vi "Vision Tracking.vi"(0 "Color Image In":T4, 1 "Score Limits":T7={"Rect Coverage"=76.0, "Aspect Ratio"=70.0, "X Edge Strength"=40.0, "Y Edge Strength"=60.0}, 3 "Decimate by":cluster{"H":i32, "V":i32}={"H"=3, "V"=5}, 4 "Color Range":T8={"Hue"={"Lower"=55, "Upper"=93}, "Sat"={"Lower"=41, "Upper"=255}, " Luma"={"Lower"=99, "Upper"=255}}, 5 "Left Offset Percentage":dbl=3.0, 6 "Camera Type":enum16{"206", "1011"}(ring), 9 "Particle Count Limit":i32=10, 11 "Display Mask":bool, 12 "Image Size":T6=enum."320x240", 13 "Area Size Limit":i32=444) -> (14 "Processed Image":T4, 15 "Distance (ft)":dbl, 17 "Target Info":T5(array[cluster]), 18 "Position.X":dbl, 19 "Center Line X":dbl)   [LabVIEW 2011]
uses:
  <vilib>/vision/Image Controls.llb/IMAQ Image.ctl
  <vilib>/Rock Robotics/WPI/Camera/WPI_CameraImageSize.ctl
  <vilib>/addons/control/pid/NI_PID_pid.lvlib
panel:
  out "Top Goal Left and Right":cluster{"Left":dbl, "Right":dbl}
  out "x+y":dbl
  out "x*y":dbl
  in  "reinitialize? (F)":bool
  out "Target Angle":dbl
  in  "saturation Gyro":dbl=0.7
  in  "PID gains Gyro":T1={"proportional gain (Kc)"=0.03, "integral time (Ti, min)"=0.01, "derivative time (Td, min)"=0.002} {"derivative time (Td, min)" format="%#.7g"; "integral time (Ti, min)" format="%#.6g"; "proportional gain (Kc)" format="%#.6g"}
  in  "Gyro Angle (deg)":dbl(knob)=3.7731857266145283 scale=-45.0..45.0
  out "Rotation":dbl=-0.26122391808015843
  out "Top Goal":T2
  out "Index":i32
  out "Top Goal":T3
  out "Min Top":dbl
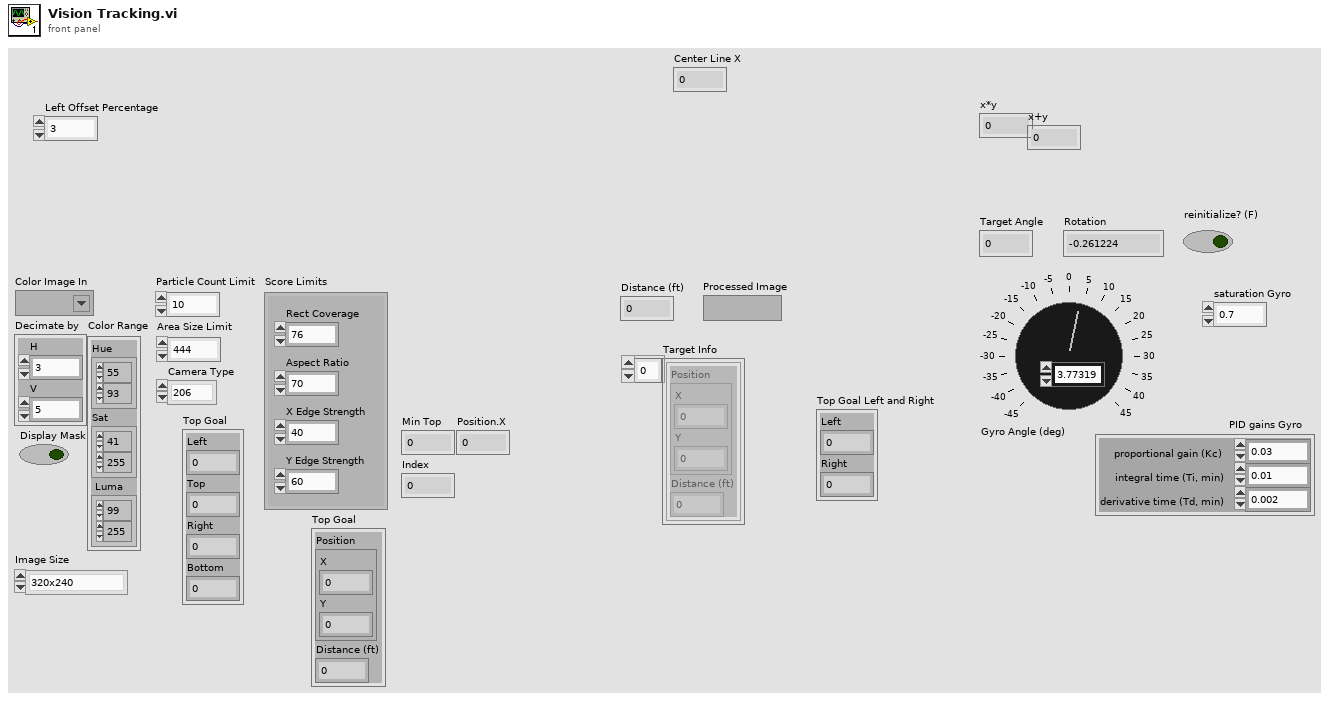
[diagram p1: front panel]
types:
  T1 = cluster{"proportional gain (Kc)":dbl, "integral time (Ti, min)":dbl, "derivative time (Td, min)":dbl}
  T2 = cluster{"Position":cluster{"X":dbl, "Y":dbl}, "Distance (ft)":dbl}
  T3 = cluster{"Left":dbl, "Top":dbl, "Right":dbl, "Bottom":dbl}
  T4 = typedef "IMAQ Image.ctl" = refnum<image>
  T5 = cluster{"Position":cluster{"X":dbl, "Y":dbl}, "Distance (ft)":dbl}[]
  T6 = typedef "WPI_CameraImageSize.ctl" = enum16{"640x480", "320x240", "160x120"}
  T7 = cluster{"Rect Coverage":dbl, "Aspect Ratio":dbl, "X Edge Strength":dbl, "Y Edge Strength":dbl}
  T8 = cluster{"Hue":cluster{"Lower":i32, "Upper":i32}, "Sat":cluster{"Lower":i32, "Upper":i32}, " Luma":cluster{"Lower":i32, "Upper":i32}}
  T9 = cluster{cluster{"Left":dbl, "Top":dbl, "Right":dbl, "Bottom":dbl}, dbl[]}[]
  T10 = cluster{"Target Center (-1 to 1)":cluster{"X":dbl, "Y":dbl}, "Distance (ft)":dbl}
  T11 = cluster{"Target Center (-1 to 1)":cluster{"X":dbl, "Y":dbl}, "Distance (ft)":dbl}[]
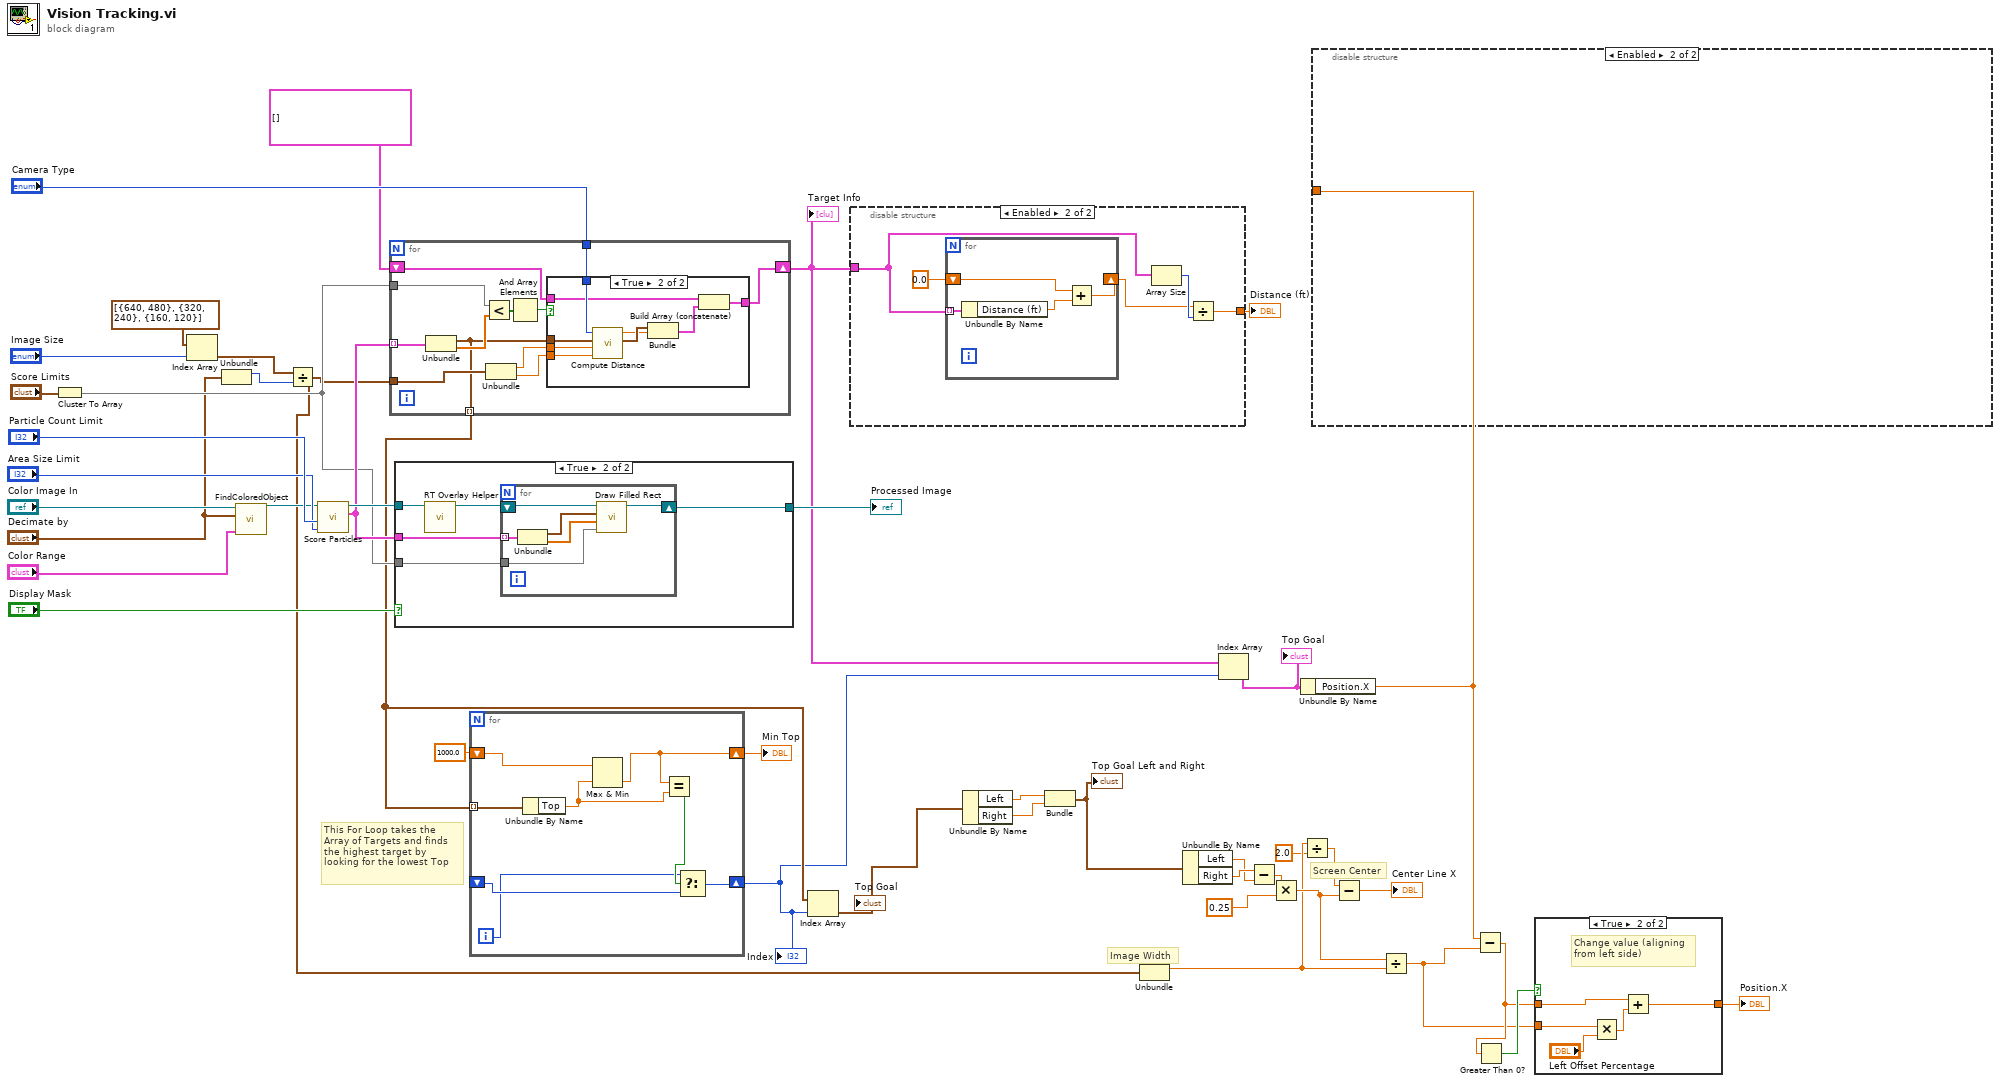
[diagram p0: block diagram]
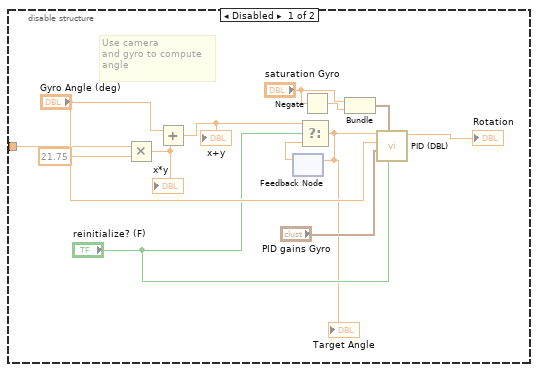
[diagram p3: hidden frame]
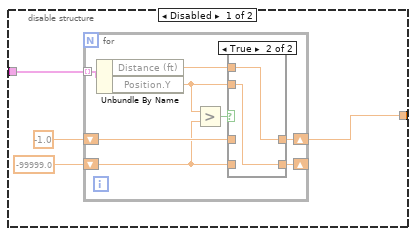
[diagram p4: hidden frame]
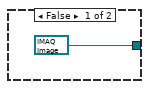
[diagram p6: hidden frame]
diagram:
  # "Screen Center"
  # "Image Width"
  # "This For Loop takes the Array of Targets and finds the highest target by looking for the lowest Top"
  n1 = Cluster To Array(cluster="Score Limits") -> (array=w32:dbl[])
  n2 = Index Array(array=cluster{i32, i32}[] [{640, 480}, {320, 240}, {160, 120}], index="Image Size") -> (element=w30:cluster{i32, i32})
  n3 = Unbundle("Decimate by") -> ("H"=w28:i32)  [unwired: 1 out]
  n4 = call "FindColoredObject.vi"("Color Range"="Color Range", "Decimate by"="Decimate by", "Color Image In"="Color Image In") -> ("Mask Image"=w40:T4)  [unwired: 3 in, 3 out]
  n5 = Divide(x=w30, y=w28) -> (x/y=w9:cluster{dbl, dbl})
  n6 = call "Score Particles.vi"("Area Size Limit"="Area Size Limit", "Particle Count Limit"="Particle Count Limit", "Image Refnum in"=w40) -> ("Scored Particle Info"=w33:T9, "Image Refnum out"=w34:T4)  [unwired: 7 in]
  n7 = for {
    tunnel: w33 -> [w56] mode=indexing
    tunnel: w32 -> [w54]
    tunnel: w9 -> [w46]
    tunnel: "Camera Type" -> [w49]
    shift-right: [w47] -> w22
    shift-left: T5 [] -> [w48]
    tunnel: [w45] -> w23 mode=indexing
    n8 = Unbundle(w56) -> (w45:T3, w55:dbl[])
    n9 = Less?(x=w54, y=w55) -> (x < y?=w53:bool[])
    n10 = Unbundle(w46) -> (w51:dbl, w50:dbl)
    n11 = And Array Elements(Boolean array=w53) -> (logical AND=w52:bool)
    n12 = case shown="True" w52 {
      tunnel: w51 -> [_ w66]
      tunnel: w50 -> [_ w65]
      tunnel: w45 -> [_ w64]
      tunnel: w49 -> [_ w63]
      tunnel: w48 -> [w57 w62]
      tunnel: [w57 w61] -> w47
      frame False {
      }
      frame True {
        n13 = call "Compute Distance.vi"("Y Image Resolution"=w65, "X Image Resolution"=w66, "Bounding Box"=w64, "Camera Type"=w63) -> ("Target Center (-1 to 1)"=w60:cluster{"X":dbl, "Y":dbl}, "Distance (ft)"=w59:dbl)  [unwired: 6 in]
        n14 = Bundle("Target Center (-1 to 1)"=w60, "Distance (ft)"=w59) -> (w58:T10)  [unwired: 1 in]
        n15 = Build Array (concatenate)(w62, w58) -> (w61:T11)
      }
    }
  }
  "Target Info" <- w22
  n16 = case shown="True" "Display Mask" {
    tunnel: w34 -> [_ w72]
    tunnel: w33 -> [_ w70]
    tunnel: w32 -> [_ w69]
    tunnel: [T4 refnum ("Refnum out") w68] -> w31
    frame False {
    }
    frame True {
      n17 = call "RT Overlay Helper.vi"("Refnum in"=w72) -> ("Refnum out"=w71:T4)  [unwired: 10 in]
      n18 = for {
        tunnel: w70 -> [w77] mode=indexing
        tunnel: w69 -> [w74]
        shift-right: [w73] -> w68
        shift-left: w71 -> [w78]
        n19 = Unbundle(w77) -> (w76:T3, w75:dbl[])
        n20 = call "Draw Filled Rect.vi"("Limits"=w74, "Scores"=w75, "Bounding Box"=w76, "image in"=w78) -> ("image out"=w73:T4)  [unwired: 7 in]
      }
    }
  }
  "Processed Image" <- w31
  n21 = for {
    shift-right: [w84] -> w24
    shift-left: 1000.0 -> [w86]
    tunnel: w23 -> [w85] mode=indexing
    shift-right: [w81] -> w21
    shift-left: _ -> [w80]
    i -> [w79]
    n22 = Unbundle By Name(w85) -> ("Top"=w82:dbl)
    n23 = Max & Min(x=w86, y=w82) -> (min(x,y)=w84:dbl)  [unwired: 1 out]
    n24 = Equal?(x=w84, y=w82) -> (x = y?=w83:bool)
    n25 = Select(t=w79, s=w83, f=w80) -> (s? t:f=w81:i32)
  }
  "Min Top" <- w24
  "Index" <- w21
  n26 = Index Array(array=w23, index=w21) -> (element=w19:T3)
  "Top Goal" <- w19
  n27 = disable-structure shown="Enabled" {
    disable-tunnel: w22 -> [w88 w107]
    disable-tunnel: [w87 w103] -> w27
    frame Disabled {
      n28 = for {
        tunnel: w88 -> [w98] mode=indexing
        shift-right: [w94] -> w87
        shift-left: -1.0 ("y") -> [w95]
        shift-right: [w96] -> _
        shift-left: -99999.0 ("y") -> [w93]
        n29 = Unbundle By Name(w98) -> ("Distance (ft)"=w92:dbl, "Position.Y"=w91:dbl)
        n30 = Greater?(x=w91, y=w93) -> (0:w97:bool)
        n31 = case shown="True" w97 {
          tunnel: w93 -> [w100 _]
          tunnel: [w100 w102] -> w96
          tunnel: [w99 w101] -> w94
          tunnel: w95 -> [w99 _]
          tunnel: w92 -> [_ w101]
          tunnel: w91 -> [_ w102]
          frame False {
          }
          frame True {
          }
        }
      }
    }
    frame Enabled {
      n32 = for {
        tunnel: w107 -> [w111] mode=indexing
        shift-right: [w109] -> w104
        shift-left: 0.0 -> [w108]
        n33 = Unbundle By Name(w111) -> ("Distance (ft)"=w110:dbl)
        n34 = Add(x=w108, y=w110) -> (x+y=w109:dbl)
      }
      n35 = Array Size(array=w107) -> (size(s)=w105:i32)
      n36 = Divide(x=w104, y=w105) -> (x/y=w103:dbl)
    }
  }
  "Distance (ft)" <- w27
  n37 = Unbundle By Name(w19) -> ("Left"=w18:dbl, "Right"=w17:dbl)
  n38 = Bundle("Left"=w18, "Right"=w17) -> (w12:cluster{"Left":dbl, "Right":dbl})  [unwired: 1 in]
  "Top Goal Left and Right" <- w12
  n39 = Unbundle(w9) -> (w7:dbl)  [unwired: 1 out]
  n40 = Unbundle By Name(w12) -> ("Left"=w15:dbl, "Right"=w16:dbl)
  n41 = Index Array(array=w22, index=w21) -> (element=w20:T2)
  "Top Goal" <- w20
  n42 = Subtract(x=w16, y=w15) -> (x-y=w14:dbl)
  n43 = Multiply(x=w14, y=0.25 ("Y")) -> (x*y=w10:dbl)
  n44 = Unbundle By Name(w20) -> ("Position.X"=w8:dbl)
  n45 = Divide(x=w7, y=2.0) -> (x/y=w5:dbl)
  n46 = disable-structure shown="Enabled" {
    disable-tunnel: w8 -> [w112 _]
    frame Disabled {
      # "Use camera\nand gyro to compute\nangle"
      n47 = Multiply(x=w112, y=sgl 21.75 ("deg full screen 2")) -> (x*y=w117:dbl)
      "x*y" <- w117
      n48 = Add(x="Gyro Angle (deg)", y=w117) -> (x+y=w115:dbl)
      "x+y" <- w115
      n49 = feedback #1() -> (w116:dbl)  [unwired: 1 out]
      n50 = Select(t=w115, s="reinitialize? (F)", f=w116) -> (s? t:f=w113:dbl)
      "Target Angle" <- w113
      n51 = feedback-in #1(w113) -> ()
      n52 = Negate(x="saturation Gyro") -> (-x=w123:dbl)
      n53 = Bundle("saturation Gyro"="saturation Gyro", w123) -> (w120:cluster{"saturation Gyro":dbl, dbl})  [unwired: 1 out]
      n54 = call <vilib>:"PID (DBL).vi"("reinitialize? (F)"="reinitialize? (F)", "output range"=w120, "PID gains"="PID gains Gyro", "process variable"="Gyro Angle (deg)", "setpoint"=w113) -> ("output"=→"Rotation":dbl)  [unwired: 1 in, 5 out]
    }
    frame Enabled {
    }
  }
  n55 = Subtract(x=w5, y=w10) -> (x-y=→"Center Line X":dbl)
  n56 = Divide(x=w10, y=w7) -> (x/y=w1:dbl)
  n57 = Subtract(x=w8, y=w1) -> (x-y=w2:dbl)
  n58 = Greater Than 0?(x=w2) -> (x > 0?=w4:bool)
  n59 = case shown="True" w4 {
    tunnel: [w125 w128] -> w3
    tunnel: w2 -> [w125 w129]
    tunnel: w1 -> [_ w130]
    frame False {
    }
    frame True {
      # "Change value (aligning\nfrom left side)"
      n60 = Multiply(x=w130, y="Left Offset Percentage") -> (x*y=w127:dbl)
      n61 = Add(x=w129, y=w127) -> (x+y=w128:dbl)
    }
  }
  "Position.X" <- w3
